vi "Test Path with No PPL Namespace.vi"(8 "error in (no error)":errorcluster, 11 "TestCase in":refnum<class "Test Configure RunTime Path.lvclass">) -> (0 "error out":errorcluster, 3 "TestCase out":refnum<class "Test Configure RunTime Path.lvclass">)   [LabVIEW 2019, in "Test Configure RunTime Path.lvclass"]
uses:
  Test Configure RunTime Path.lvclass
  C:/Program Files/National Instruments/LabVIEW 2024/vi.lib/Astemes/LUnit/Test Case.lvclass
  <vilib>/Astemes/LUnit/Test Case.lvclass/Test Case.ctl
  829fd33e-19ac-4a12-9731-6f80797580f2.vi
  <vilib>/Astemes/LUnit/Core/LUnit Test Case/Private/Append Pass Result.vi
  <vilib>/Astemes/LUnit/Core/LUnit Test Case/Private/Append Fail Result.vi
  829fd33e-19ac-4a12-9731-6f80797580f2.vi/9c5d11cd-9439-4240-a1ee-d9baace9c924.vi
  <vilib>/Astemes/LUnit/Core/LUnit Test Case/Private/Run In UI.vi
  <vilib>/Utility/error.llb/Clear Errors.vi
  TSC File IO.lvlib
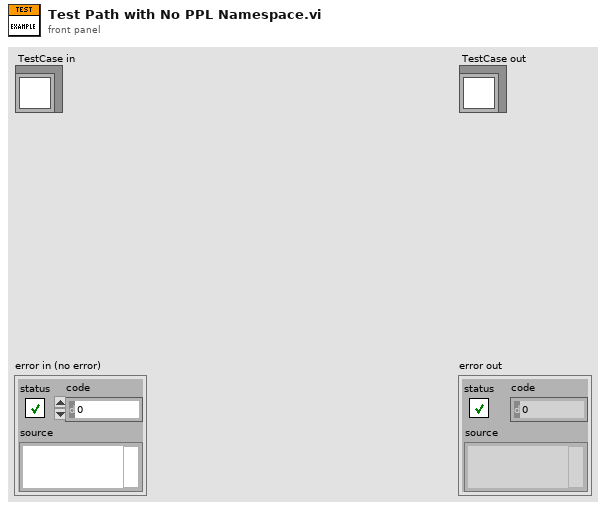
[diagram p1: front panel]
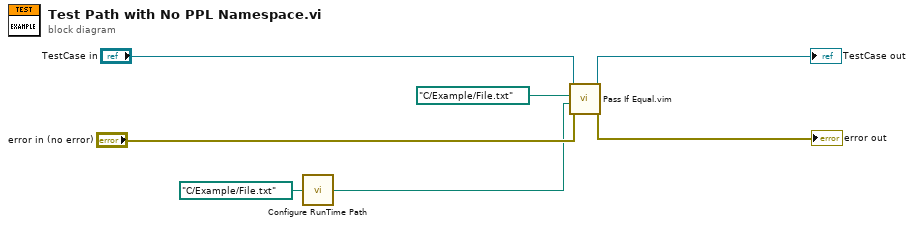
[diagram p0: block diagram]
diagram:
  n1 = call "Configure RunTime Path.vi"("Input Path"=path "C:/Example/File.txt") -> ("Updated Path"=w2:path)
  n2 = call "Pass If Equal.vim"("error in (no error)"="error in (no error)", "Actual"=w2, "Expected"=path "C:/Example/File.txt", "LUnit Test Case In"="TestCase in") -> ("error out"=→"error out":errorcluster, "LUnit Test Case Out"=→"TestCase out":refnum<class "Test Configure RunTime Path.lvclass">)  [unwired: 6 in]
